vi "DIO Setup.vi"   [LabVIEW 2020]
uses:
  <vilib>/Rock Robotics/SystemInterfaces/DIO/FPGA_DIOChannel.ctl
types:
  T1 = typedef "FPGA_DIOChannel.ctl" = enum8{"DIO 0", "DIO 1", "DIO 2", "DIO 3", "DIO 4", "DIO 5", "DIO 6", "DIO 7", "DIO 8", "DIO 9", "DIO MXP 0", "DIO MXP 1", "DIO MXP 2", "DIO MXP 3", "DIO MXP 4", "DIO MXP 5", "DIO MXP 6", "DIO MXP 7", "DIO MXP 8", "DIO MXP 9", "DIO MXP 10", "DIO MXP 11", "DIO MXP 12", "DIO MXP 13", "DIO MXP 14", "DIO MXP 15", "SPI Port CS1", "SPI Port CS2", "SPI Port CS3", "SPI Port MISO", "SPI Port MOSI", "Invalid"}
  T2 = typedef "WPI_DigitalInputDevRef.ctl" = cluster{"DevStatus":errorcluster, "DIO Channel":T1}
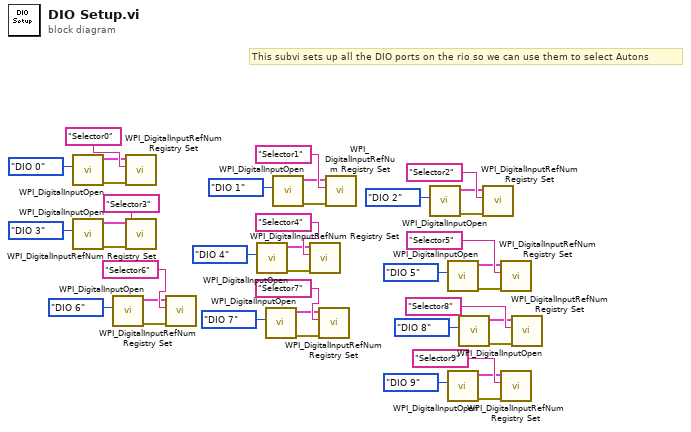
[diagram p0: block diagram]
diagram:
  # "This subvi sets up all the DIO ports on the rio so we can use them to select Autons"
  n1 = call <vilib>:"WPI_DigitalInputOpen.vi"("DIO Channel"=FPGA_DIOChannel."DIO 0") -> ("error out"=w1:errorcluster, "DigitalInputDevRef"=w2:T2)  [unwired: 9 in]
  n2 = call <vilib>:"WPI_DigitalInputOpen.vi"("DIO Channel"=FPGA_DIOChannel."DIO 3") -> ("error out"=w5:errorcluster, "DigitalInputDevRef"=w6:T2)  [unwired: 9 in]
  n3 = call <vilib>:"WPI_DigitalInputOpen.vi"("DIO Channel"=FPGA_DIOChannel."DIO 6") -> ("error out"=w8:errorcluster, "DigitalInputDevRef"=w9:T2)  [unwired: 9 in]
  n4 = call <vilib>:"WPI_DigitalInputRefNum Registry Set.vi"("error in (no error)"=w1, "refnum name"="Selector0", "DigitalInputDevRef"=w2) -> ()  [unwired: 7 in, 2 out]
  n5 = call <vilib>:"WPI_DigitalInputRefNum Registry Set.vi"("error in (no error)"=w5, "refnum name"="Selector3", "DigitalInputDevRef"=w6) -> ()  [unwired: 7 in, 2 out]
  n6 = call <vilib>:"WPI_DigitalInputRefNum Registry Set.vi"("error in (no error)"=w8, "refnum name"="Selector6", "DigitalInputDevRef"=w9) -> ()  [unwired: 7 in, 2 out]
  n7 = call <vilib>:"WPI_DigitalInputOpen.vi"("DIO Channel"=FPGA_DIOChannel."DIO 4") -> ("error out"=w14:errorcluster, "DigitalInputDevRef"=w15:T2)  [unwired: 9 in]
  n8 = call <vilib>:"WPI_DigitalInputOpen.vi"("DIO Channel"=FPGA_DIOChannel."DIO 7") -> ("error out"=w11:errorcluster, "DigitalInputDevRef"=w12:T2)  [unwired: 9 in]
  n9 = call <vilib>:"WPI_DigitalInputOpen.vi"("DIO Channel"=FPGA_DIOChannel."DIO 1") -> ("error out"=w17:errorcluster, "DigitalInputDevRef"=w18:T2)  [unwired: 9 in]
  n10 = call <vilib>:"WPI_DigitalInputRefNum Registry Set.vi"("error in (no error)"=w14, "refnum name"="Selector4", "DigitalInputDevRef"=w15) -> ()  [unwired: 7 in, 2 out]
  n11 = call <vilib>:"WPI_DigitalInputRefNum Registry Set.vi"("error in (no error)"=w11, "refnum name"="Selector7", "DigitalInputDevRef"=w12) -> ()  [unwired: 7 in, 2 out]
  n12 = call <vilib>:"WPI_DigitalInputRefNum Registry Set.vi"("error in (no error)"=w17, "refnum name"="Selector1", "DigitalInputDevRef"=w18) -> ()  [unwired: 7 in, 2 out]
  n13 = call <vilib>:"WPI_DigitalInputOpen.vi"("DIO Channel"=FPGA_DIOChannel."DIO 2") -> ("error out"=w20:errorcluster, "DigitalInputDevRef"=w21:T2)  [unwired: 9 in]
  n14 = call <vilib>:"WPI_DigitalInputOpen.vi"("DIO Channel"=FPGA_DIOChannel."DIO 5") -> ("error out"=w23:errorcluster, "DigitalInputDevRef"=w24:T2)  [unwired: 9 in]
  n15 = call <vilib>:"WPI_DigitalInputOpen.vi"("DIO Channel"=FPGA_DIOChannel."DIO 9") -> ("error out"=w29:errorcluster, "DigitalInputDevRef"=w30:T2)  [unwired: 9 in]
  n16 = call <vilib>:"WPI_DigitalInputOpen.vi"("DIO Channel"=FPGA_DIOChannel."DIO 8") -> ("error out"=w26:errorcluster, "DigitalInputDevRef"=w27:T2)  [unwired: 9 in]
  n17 = call <vilib>:"WPI_DigitalInputRefNum Registry Set.vi"("error in (no error)"=w20, "refnum name"="Selector2", "DigitalInputDevRef"=w21) -> ()  [unwired: 7 in, 2 out]
  n18 = call <vilib>:"WPI_DigitalInputRefNum Registry Set.vi"("error in (no error)"=w23, "refnum name"="Selector5", "DigitalInputDevRef"=w24) -> ()  [unwired: 7 in, 2 out]
  n19 = call <vilib>:"WPI_DigitalInputRefNum Registry Set.vi"("error in (no error)"=w29, "refnum name"="Selector9", "DigitalInputDevRef"=w30) -> ()  [unwired: 7 in, 2 out]
  n20 = call <vilib>:"WPI_DigitalInputRefNum Registry Set.vi"("error in (no error)"=w26, "refnum name"="Selector8", "DigitalInputDevRef"=w27) -> ()  [unwired: 7 in, 2 out]
